vi "Utility_Strip_and_Replace_File_Suffix.vi"(3 "New File Suffix IN":string, 5 "File Name":string) -> (0 "Old File Suffix OUT":string, 2 "File Name":string)   [LabVIEW 2021]
doc: "This VI will strip the suffix off of a filename. The suffix is defined as any characters coming after the last period (.) in a file name.\n\nIf the \"New File Suffix IN\" control is wired, the filename will be appended with the new suffix. If it is not wired, or is an empty string, the old suffix will be stripped and the base file name will be passed out.\n\nDeveloped by:\nGreg Sussman\nProcess Automation Corp\nwww.processauto.com\n(267)685-1249"
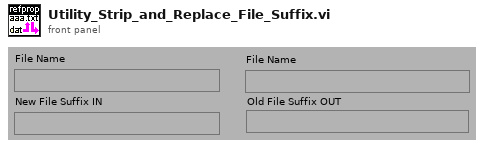
[diagram p1: front panel]
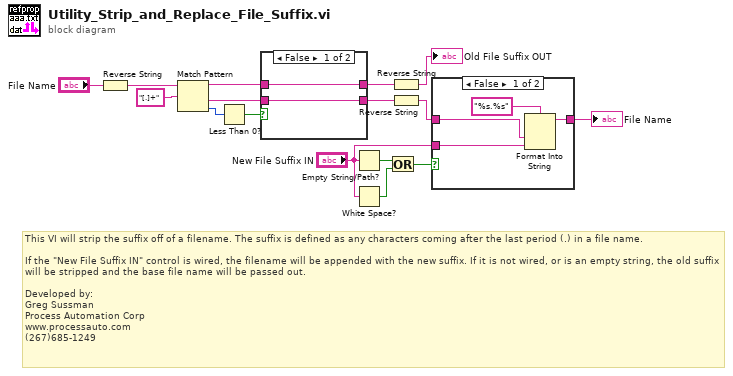
[diagram p0: block diagram]
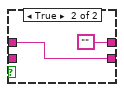
[diagram p3: hidden frame]
diagram:
  # "This VI will strip the suffix off of a filename. The suffix is defined as any characters coming after the last period (.) in a file name.\n\nIf the \"New File Suffix IN\" control is wired, the filename will be appended with the new suffix. If it is not wired, or is an empty string, the old suffix will be stripped and the base file name will be passed out.\n\nDeveloped by:\nGreg Sussman\nProcess Automation Corp\nwww.processauto.com\n(267)685-1249"
  n1 = Reverse String(1:"File Name") -> (0:w15:string)
  n2 = Match Pattern(string=w15, regular expression="[.]+") -> (before substring=w8:string, after substring=w10:string, offset past match=w13:i32)  [unwired: 1 in, 1 out]
  n3 = Less Than 0?(x=w13) -> (x < 0?=w12:bool)
  n4 = case shown="False" w12 {
    tunnel: [w18 ""] -> w11
    tunnel: w10 -> [w17 _]
    tunnel: [w17 w19] -> w9
    tunnel: w8 -> [w18 w19]
    frame False {
    }
    frame True {
    }
  }
  n5 = Empty String/Path?(string/path="New File Suffix IN") -> (empty?=w6:bool)
  n6 = White Space?(1:"New File Suffix IN") -> (0:w5:bool)
  n7 = Or(x=w6, y=w5) -> (x .or. y?=w4:bool)
  n8 = Reverse String(1:w11) -> (0:→"Old File Suffix OUT":string)
  n9 = Reverse String(1:w9) -> (0:w3:string)
  n10 = case shown="False" w4 {
    tunnel: w3 -> [w22 w25]
    tunnel: [w23 w25] -> w2
    tunnel: "New File Suffix IN" -> [w21 _]
    frame False {
      n11 = Format Into String(format string="%s.%s", w22, w21) -> (resulting string=w23:string)  [unwired: 2 in, 1 out]
    }
    frame True {
    }
  }
  "File Name" <- w2
